vi "ABB Extract entries.vi"(7 "Pulldown text":bool, 9 "Entry IDs":string[](array[string]), 10 "Entry ID":string, 11 "Entry table in":string[][](array[string])) -> (3 "Selected Entries":string[](array[string]))   [LabVIEW 2017]
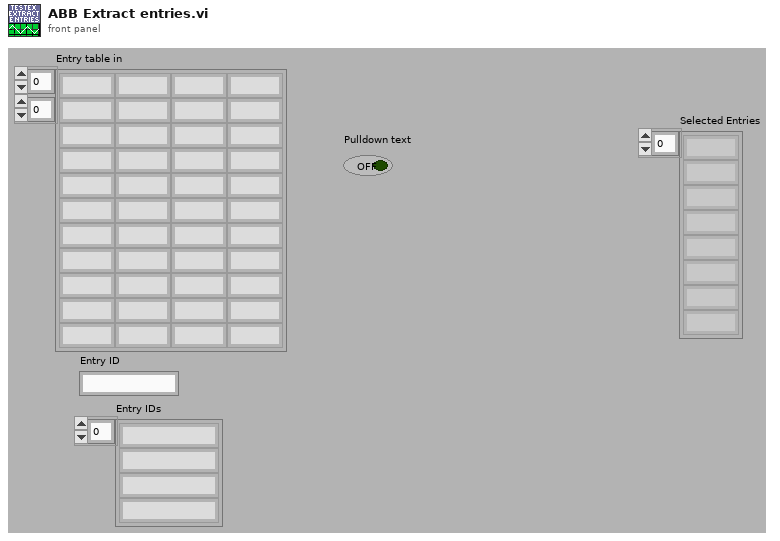
[diagram p1: front panel]
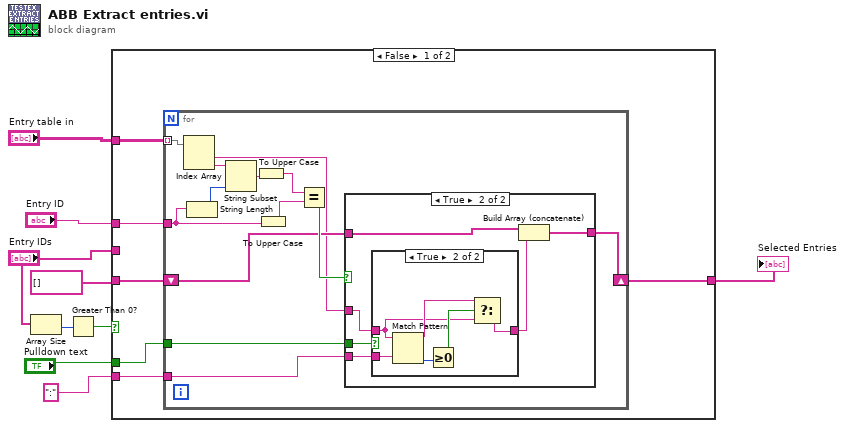
[diagram p0: block diagram]
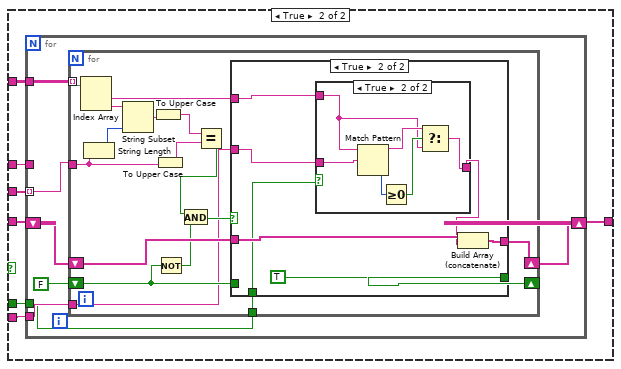
[diagram p4: hidden frame]
diagram:
  n1 = Array Size(array="Entry IDs") -> (size(s)=w5:i32)
  n2 = Greater Than 0?(x=w5) -> (x > 0?=w4:bool)
  n3 = case shown="False" w4 {
    tunnel: "Entry table in" -> [w15 w49]
    tunnel: "Entry ID" -> [w14 w48]
    tunnel: string[] [] -> [w13 w46]
    tunnel: [w12 w47] -> w6
    tunnel: "Entry IDs" -> [_ w45]
    tunnel: "Pulldown text" -> [w11 w43]
    tunnel: ":" -> [w10 w44]
    frame False {
      n4 = for {
        tunnel: w15 -> [w28] mode=indexing
        tunnel: w14 -> [w18]
        shift-right: [w20] -> w12
        shift-left: w13 -> [w22]
        tunnel: w11 -> [w17]
        tunnel: w10 -> [w16]
        n5 = Index Array(array=w28) -> (element #1=w21:string, element #2=w27:string)  [unwired: 2 in]
        n6 = String Length(string=w18) -> (length=w19:i32)
        n7 = String Subset(string=w27, length (rest)=w19) -> (substring=w26:string)  [unwired: 1 in]
        n8 = To Upper Case(1:w26) -> (0:w25:string)
        n9 = To Upper Case(1:w18) -> (0:w24:string)
        n10 = Equal?(x=w25, y=w24) -> (x = y?=w23:bool)
        n11 = case shown="True" w23 {
          tunnel: w22 -> [w29 w35]
          tunnel: w21 -> [_ w32]
          tunnel: [w29 w34] -> w20
          tunnel: w17 -> [_ w33]
          tunnel: w16 -> [_ w30]
          frame False {
          }
          frame True {
            n12 = case shown="True" w33 {
              tunnel: w32 -> [w36 w37]
              tunnel: [w36 w38] -> w31
              tunnel: w30 -> [_ w42]
              frame False {
              }
              frame True {
                n13 = Match Pattern(string=w37, regular expression=w42) -> (before substring=w39:string, offset past match=w41:i32)  [unwired: 1 in, 2 out]
                n14 = Greater Or Equal To 0?(x=w41) -> (x >= 0?=w40:bool)
                n15 = Select(t=w39, s=w40, f=w37) -> (s? t:f=w38:string)
              }
            }
            n16 = Build Array (concatenate)(w35, w31) -> (w34:string[])
          }
        }
      }
    }
    frame True {
      n17 = for {
        tunnel: w49 -> [w56]
        tunnel: w48 -> [_]
        shift-right: [w55] -> w47
        shift-left: w46 -> [w54]
        tunnel: w45 -> [w53] mode=indexing
        tunnel: w44 -> [w51]
        tunnel: w43 -> [w50]
        n18 = for {
          tunnel: w56 -> [w73] mode=indexing
          tunnel: w53 -> [w64]
          shift-right: [w66] -> w55
          shift-left: w54 -> [w67]
          shift-right: [w63] -> _
          shift-left: FALSE -> [w62]
          tunnel: w51 -> [w58]
          tunnel: w50 -> [w57]
          n19 = Index Array(array=w73) -> (element #1=w59:string, element #2=w72:string)  [unwired: 2 in]
          n20 = String Length(string=w64) -> (length=w65:i32)
          n21 = String Subset(string=w72, length (rest)=w65) -> (substring=w71:string)  [unwired: 1 in]
          n22 = To Upper Case(1:w71) -> (0:w70:string)
          n23 = To Upper Case(1:w64) -> (0:w69:string)
          n24 = Not(x=w62) -> (.not. x?=w60:bool)
          n25 = Equal?(x=w70, y=w69) -> (x = y?=w68:bool)
          n26 = And(x=w68, y=w60) -> (x .and. y?=w61:bool)
          n27 = case shown="True" w61 {
            tunnel: w67 -> [w75 w82]
            tunnel: [w75 w81] -> w66
            tunnel: w62 -> [w74 _]
            tunnel: [w74 TRUE] -> w63
            tunnel: w59 -> [_ w79]
            tunnel: w58 -> [_ w77]
            tunnel: w57 -> [_ w76]
            frame False {
            }
            frame True {
              n28 = case shown="True" w76 {
                tunnel: w79 -> [w83 w85]
                tunnel: [w83 w84] -> w78
                tunnel: w77 -> [_ w89]
                frame False {
                }
                frame True {
                  n29 = Match Pattern(string=w85, regular expression=w89) -> (before substring=w86:string, offset past match=w88:i32)  [unwired: 1 in, 2 out]
                  n30 = Greater Or Equal To 0?(x=w88) -> (x >= 0?=w87:bool)
                  n31 = Select(t=w86, s=w87, f=w85) -> (s? t:f=w84:string)
                }
              }
              n32 = Build Array (concatenate)(w82, w78) -> (w81:string[])
            }
          }
        }
      }
    }
  }
  "Selected Entries" <- w6
